vi "Display Hinter.vi"(8 "error in (no error)":errorcluster, 10 "Hint Ref":refnum<vi>, 11 "Member_Actor in":refnum<class "Member_Actor.lvclass">) -> (0 "error out":errorcluster, 3 "Member_Actor out":refnum<class "Member_Actor.lvclass">)   [LabVIEW 2015, in "Member_Actor.lvlib" / "Member_Actor.lvclass"]
uses:
  Member_Actor.lvclass
  Member_Actor.lvclass/Member_Actor.ctl
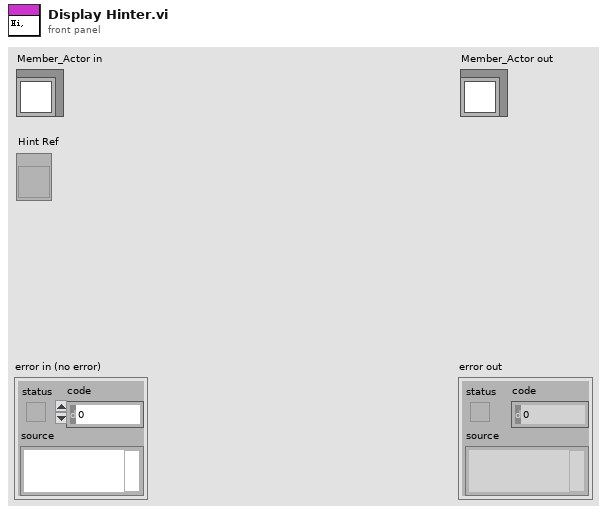
[diagram p1: front panel]
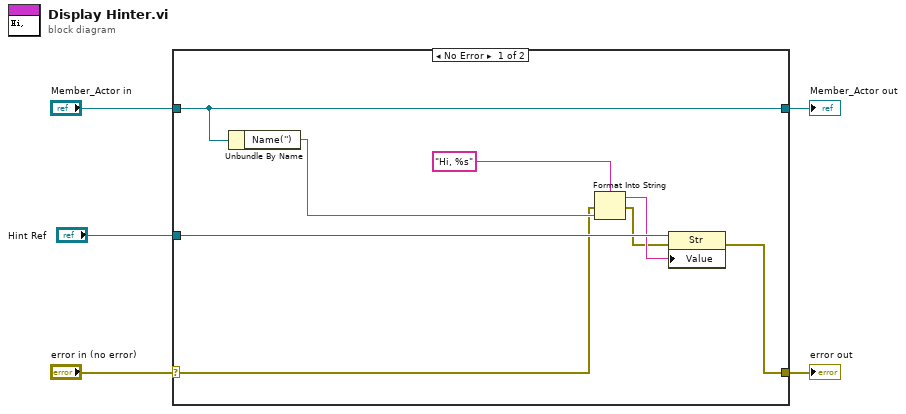
[diagram p0: block diagram]
diagram:
  n1 = case shown="No Error" "error in (no error)" {
    selector: "error in (no error)" -> [w6 w15]
    tunnel: [w8 w15] -> w4
    tunnel: [w13 w14] -> w2
    tunnel: "Member_Actor in" -> [w13 w14]
    tunnel: "Hint Ref" -> [w11 _]
    frame No Error {
      n2 = Unbundle By Name(w13) -> ("Name('')"=w7:string)
      n3 = Format Into String(format string="Hi, %s", error in=w6, w7) -> (resulting string=w10:string, error out=w9:errorcluster)  [unwired: 1 in]
      n4 = property class="Str"(reference=w11, error in=w9, "Value"=w10) -> (error out=w8:errorcluster)  [unwired: 1 out]
    }
    frame Error {
    }
  }
  "error out" <- w4
  "Member_Actor out" <- w2
